vi "APS load param from file.vi"(8 "error in (no error)":errorcluster caption="错误输入（无错误）", 11 "pXMLFile":string) -> (0 "error out":errorcluster caption="错误输出", 3 "function return":i32)   [LabVIEW 2017]
doc: "I32 FNTYPE APS_load_param_from_file( const char *pXMLFile );"
uses:
  APS168.dll
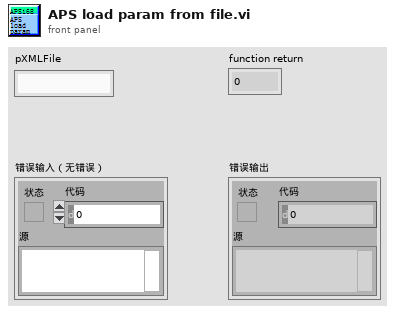
[diagram p1: front panel]
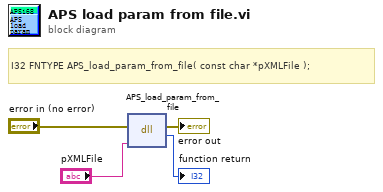
[diagram p0: block diagram]
diagram:
  # "I32 FNTYPE APS_load_param_from_file( const char *pXMLFile );"
  n1 = dll-call lib="PTH2Gabs E迈治LV范例testSubVIsADLINKMotion204cAPS168.*" fn="APS_load_param_from_file"(error in="error in (no error)", "pXMLFile"="pXMLFile") -> (error out=→"error out":errorcluster, →"function return":i32)  [unwired: 3 in, 1 out]
